vi "污染物CP编码.vi"(5 "地表水/污染源":bool, 6 "字符串":string="N", 7 "字段结束":bool=TRUE, 8 "数据类型":string(combo)="-Rtd=", 9 "污染物浓度":string, 10 "污染物编码":string) -> (3 "编码输出":string)   [LabVIEW 2016, in "数据传输系统.lvlib"]
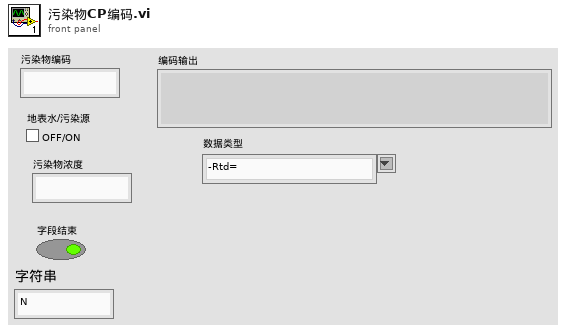
[diagram p1: front panel]
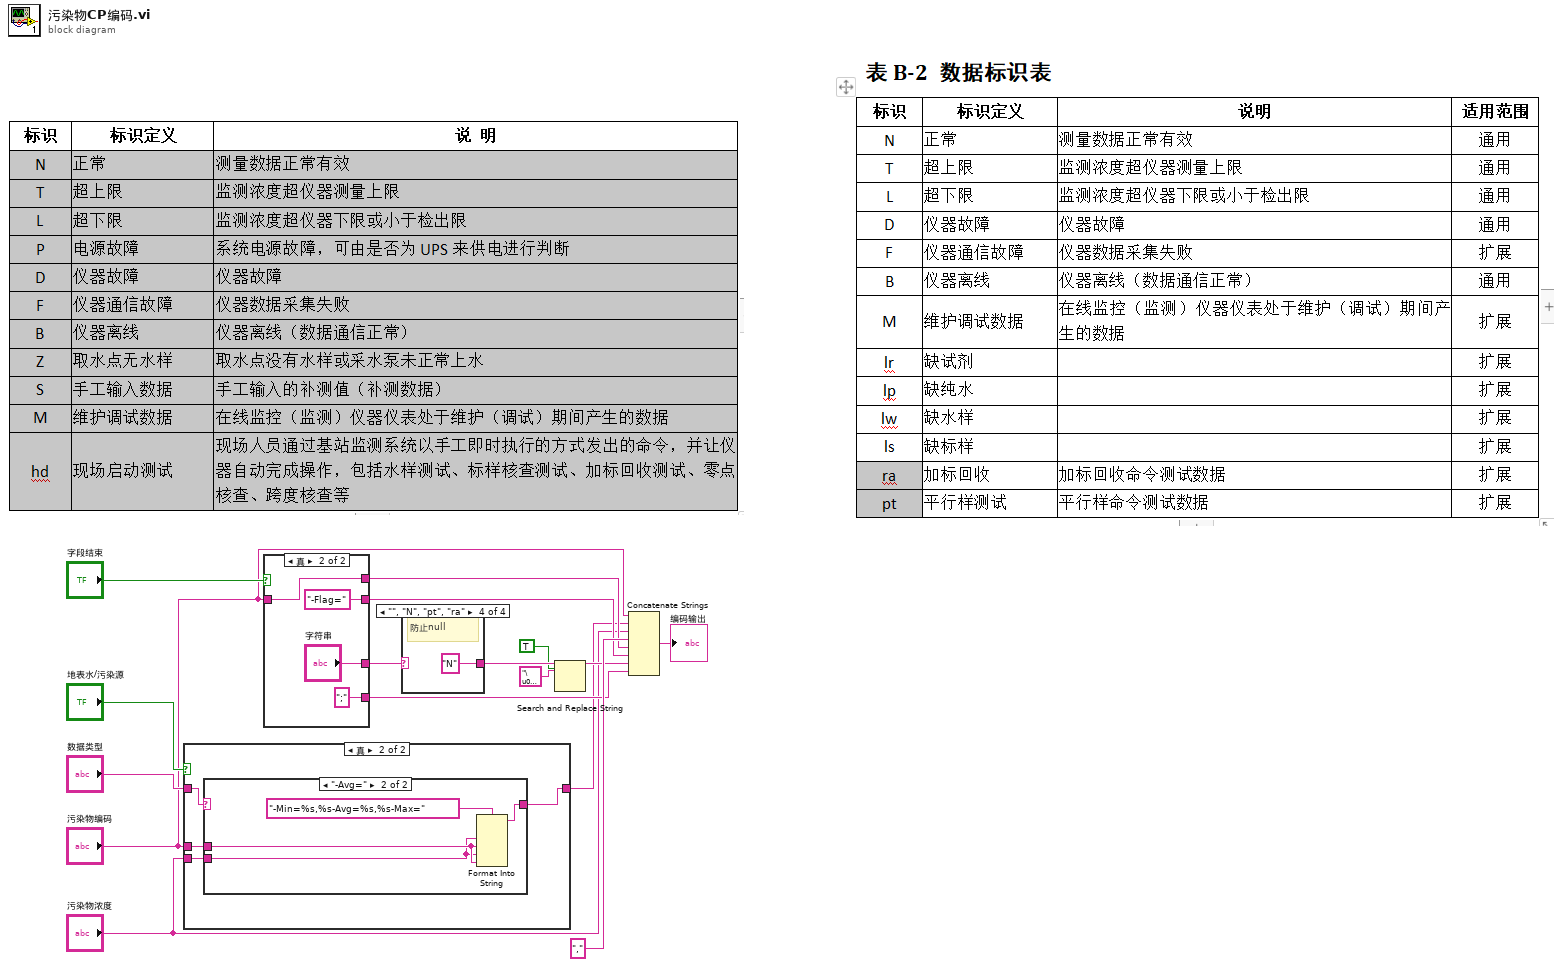
[diagram p0: block diagram]
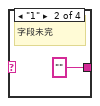
[diagram p5: hidden frame]
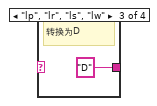
[diagram p6: hidden frame]
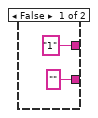
[diagram p7: hidden frame]
diagram:
  n1 = case shown="真" "地表水/污染源" {
    tunnel: "数据类型" -> [w17 w21]
    tunnel: [w17 w20] -> w2
    tunnel: "污染物编码" -> [_ w19]
    tunnel: "污染物浓度" -> [_ w18]
    frame False {
    }
    frame True {
      n2 = case shown="\"-Avg=\"" w21 {
        selector: w21 -> [w22 _]
        tunnel: [w22 w23] -> w20
        tunnel: w19 -> [_ w25]
        tunnel: w18 -> [_ w24]
        frame "假", Default {
        }
        frame "-Avg=" {
          n3 = Format Into String(format string="-Min=%s,%s-Avg=%s,%s-Max=" ("格式字符串"), w24, w25, w24, w25) -> (resulting string=w23:string)  [unwired: 2 in, 1 out]
        }
      }
    }
  }
  n4 = case shown="真" "字段结束" {
    tunnel: [_ "-Flag=" ("字符串")] -> w14
    tunnel: ["1" ("字符串") "字符串"] -> w11
    tunnel: "污染物编码" -> [_ w31]
    tunnel: [_ w31] -> w12
    tunnel: ["" ("字符串") ";" ("字符串")] -> w6
    frame False {
    }
    frame True {
    }
  }
  n5 = case shown="\"\", \"N\", \"pt\", \"ra\"" w11 {
    selector: w11 -> [w33 _ _ _]
    tunnel: [w33 "" ("字符串") "D" ("字符串") "N" ("字符串")] -> w10
    frame Default {
      # "其他透传"
    }
    frame "1" {
      # "字段未完"
    }
    frame "lp", "lr", "ls", "lw" {
      # "转换为D"
    }
    frame "", "N", "pt", "ra" {
      # "防止null"
    }
  }
  n6 = Search and Replace String(replace all?=TRUE ("替换全部？(F)"), input string=w10, search string="\u0000" ("搜索字符串")) -> (result string=w8:string)  [unwired: 5 in, 3 out]
  n7 = Concatenate Strings("污染物编码", w2, "污染物浓度", "," ("字符串"), w12, w14, w8, w6) -> (→"编码输出":string)
